vi "Target VI Write.vi"(4 "error in (no error)":errorcluster, 5 "Value":path, 6 "Container State":T2, 7 "Display State In":T1) -> (0 "error out":errorcluster, 3 "Display State Out":T1)   [LabVIEW 2009, in "Jump Button (System).xctl"]
uses:
  <vilib>/Navigation Controls/Jump Button System/Jump Button (System).xctl
  <vilib>/_xctls/Container State.ctl
  <vilib>/Navigation Controls/Jump Button System/Jump Button State.ctl
  <vilib>/_xctls/XControlSupport.lvlib
panel:
  # "Replace the Value Control below with a Control of desired type.\nDo not remove this Control or the others from the connector pane.\nDo not change the connector pane pattern.\nThe Value control should always be the third terminal from top on the input side in the connector pane."
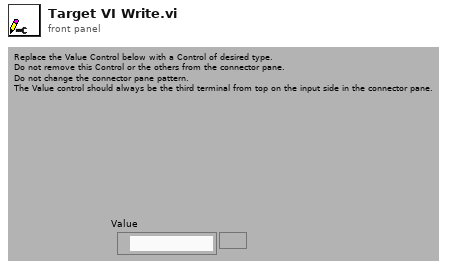
[diagram p1: front panel]
types:
  T1 = typedef "Jump Button (System).xctl/Jump Button State.ctl" = cluster{"Button Text":string, "Absolute Path":path, "Relative Path":path}
  T2 = typedef "XControlSupport.lvlib/Container State.ctl" = cluster{"Indicator?":bool, "Run Mode?":bool, " Refnum":refnum<vi>}
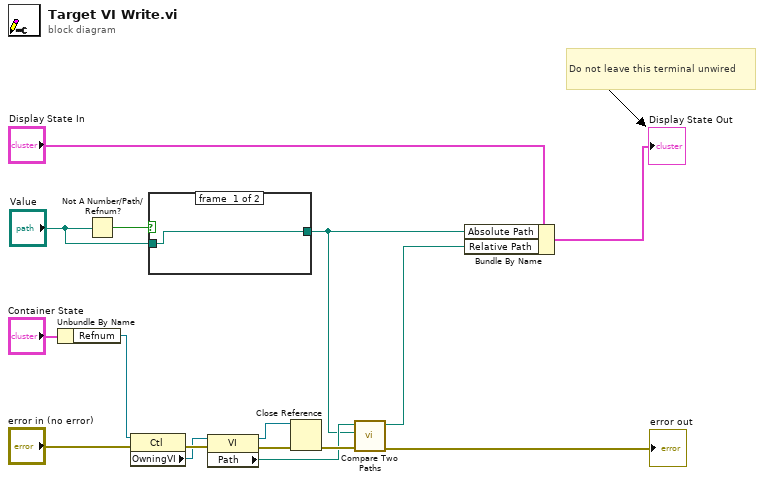
[diagram p0: block diagram]
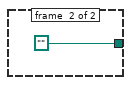
[diagram p2: hidden frame]
diagram:
  # "Do not leave this terminal unwired"
  n1 = Unbundle By Name("Container State") -> ("Refnum"=w16:refnum<vi>)
  n2 = Not A Number/Path/Refnum?(number/path/refnum="Value") -> (NaN/Path/Refnum?=w9:bool)
  n3 = property class="Ctl"(reference=w16, error in="error in (no error)") -> (error out=w15:errorcluster, "OwningVI"=w14:refnum<vi>)  [unwired: 1 out]
  n4 = case shown="False" w9 {
    tunnel: [w17 path ""] -> w8
    tunnel: "Value" -> [w17 _]
    frame #0 {
    }
    frame #1 {
    }
  }
  n5 = property class="VI"(reference=w14, error in=w15) -> (reference out=w12:refnum<vi>, error out=w13:errorcluster, "Path"=w10:path)
  n6 = Close Reference(reference=w12, error in (no error)=w13) -> (error out=w11:errorcluster)
  n7 = call <vilib>:"Compare Two Paths.vi"("error in (no error)"=w11, "Path 2"=w8, "Path 1"=w10) -> ("error out"=→"error out":errorcluster, "Relative Path from 1 to 2"=w7:path)  [unwired: 5 in, 2 out]
  n8 = Bundle By Name(cluster="Display State In", "Absolute Path"=w8, "Relative Path"=w7) -> (→"Display State Out":T1)
